vi "Configure.vi"(8 "error in":errorcluster, 10 "name":string="ePAS", 11 "ePAS in":refnum<class "ePAS.lvclass">) -> (0 "error out":errorcluster, 3 "ePAS out":refnum<class "ePAS.lvclass">)   [LabVIEW 2018, in "ePAS Library.lvlib" / "ePAS.lvclass"]
doc: "Configure the instrument class. If there is no config file specified, an error"
uses:
  ePAS.lvclass
  C:/Users/Labview/Documents/exscalabar_server/reusable/Instrument/Instrument.lvclass
  FPGA/Session/Exscalabar FPGA.lvclass
  C:/Program Files (x86)/National Instruments/LabVIEW 2018/user.lib/_Session Fwk/Session - Root.lvclass
  Commands/Change Laser Voffset/Change Laser Voffset.lvclass
  C:/Users/Labview/Documents/exscalabar_server/reusable/Command/Command.lvclass
  Commands/Change Laser Modulation/Change Laser Modulation.lvclass
  Commands/Change Laser Vrange/Change Laser Vrange.lvclass
  Commands/Change PAS Laser Frequency/Change Laser Frequency.lvclass
  Commands/Change Speaker State/Change Speaker State.lvclass
  Commands/Change Speaker Switch State/Change Speaker Switch State.lvclass
  Commands/Change iSpk Signal/Change iSpk Signal.lvclass
  Commands/Change Speaker Vparams/Change Speaker Vparams.lvclass
  Commands/Copy of Change Laser Enable State/Change Laser Enable State.lvclass
  reusable/Instrument/Instrument.lvclass/Instrument.ctl
  ePAS.lvclass/ePAS.ctl
  FPGA/Session/Exscalabar FPGA.lvclass/Exscalabar FPGA.ctl
  reusable/Session APIs/File Access/Config Data/Config Data.lvclass/Config Data.ctl
  Commands/Change Laser Voffset/Change Laser Voffset.lvclass/Change Laser Voffset.ctl
  Commands/Change Laser Vrange/Change Laser Vrange.lvclass/Change Laser Vrange.ctl
  Commands/Change PAS Laser Frequency/Change Laser Frequency.lvclass/Change Laser Frequency.ctl
  Commands/Copy of Change Laser Enable State/Change Laser Enable State.lvclass/Change Laser Enable State.ctl
  Commands/Change iSpk Signal/Change iSpk Signal.lvclass/Change iSpk Signal.ctl
  Commands/Change Speaker Switch State/Change Speaker Switch State.lvclass/Change Speaker Switch State.ctl
  Commands/Change Speaker Vparams/Change Speaker Vparams.lvclass/Change Speaker Vparams.ctl
  Commands/Change Laser Modulation/Change Laser Modulation.lvclass/Change Laser Modulation.ctl
  reusable/Session APIs/File Access/Config Data/Accessors/Read Ref.vi
  reusable/Instrument/Read Log Session.vi
  reusable/Instrument/Read Cfg Session.vi
  reusable/Instrument/Read CMD.vi
  Commands/Change Speaker Switch State/Write Length.vi
  Commands/Change Speaker Switch State/Write Period.vi
  Commands/Change Speaker Switch State/Write Cycle.vi
  FPGA/Session/Write logSession.vi
  FPGA/Session/Write configSession.vi
  reusable/Session APIs/File Access/Config Data/Config Data.lvclass
  reusable/Session APIs/File Access/Config Data/Read Array/Read Boolean Array.vi
  reusable/Session APIs/File Access/Config Data/Read Array/Read DBL Array.vi
  reusable/Session APIs/File Access/Config Data/Read Array/Read String Array.vi
  <vilib>/Utility/config.llb/Read Key (Boolean).vi
  <vilib>/Utility/config.llb/Read Key (I32).vi
  <vilib>/Utility/config.llb/Read Key (Double).vi
  reusable/PAS/Main/PAS.lvclass
  <userlib>/_Session Fwk/Session - Root.lvclass
  reusable/Command/Command.lvclass
  reusable/Session APIs/Session Log/System Log.lvclass
  <vilib>/Utility/config.llb/NI_LVConfig.lvlib
  <resource>/objmgr/daqmx.rc
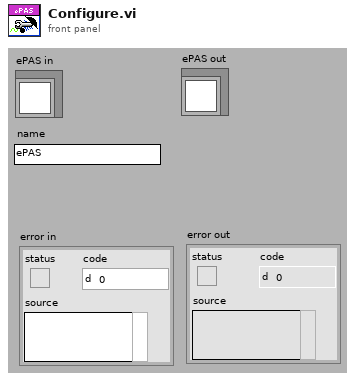
[diagram p1: front panel]
types:
  T1 = typedef "Session - Root.lvclass/Session Handle.ctl" = refnum<data-value>
  T2 = typedef "Config Data.lvclass/Config Session.ctl" = refnum<data-value>
  T3 = typedef "NI_LVConfig.lvlib/Config Data RefNum.ctl" = refnum<k1>
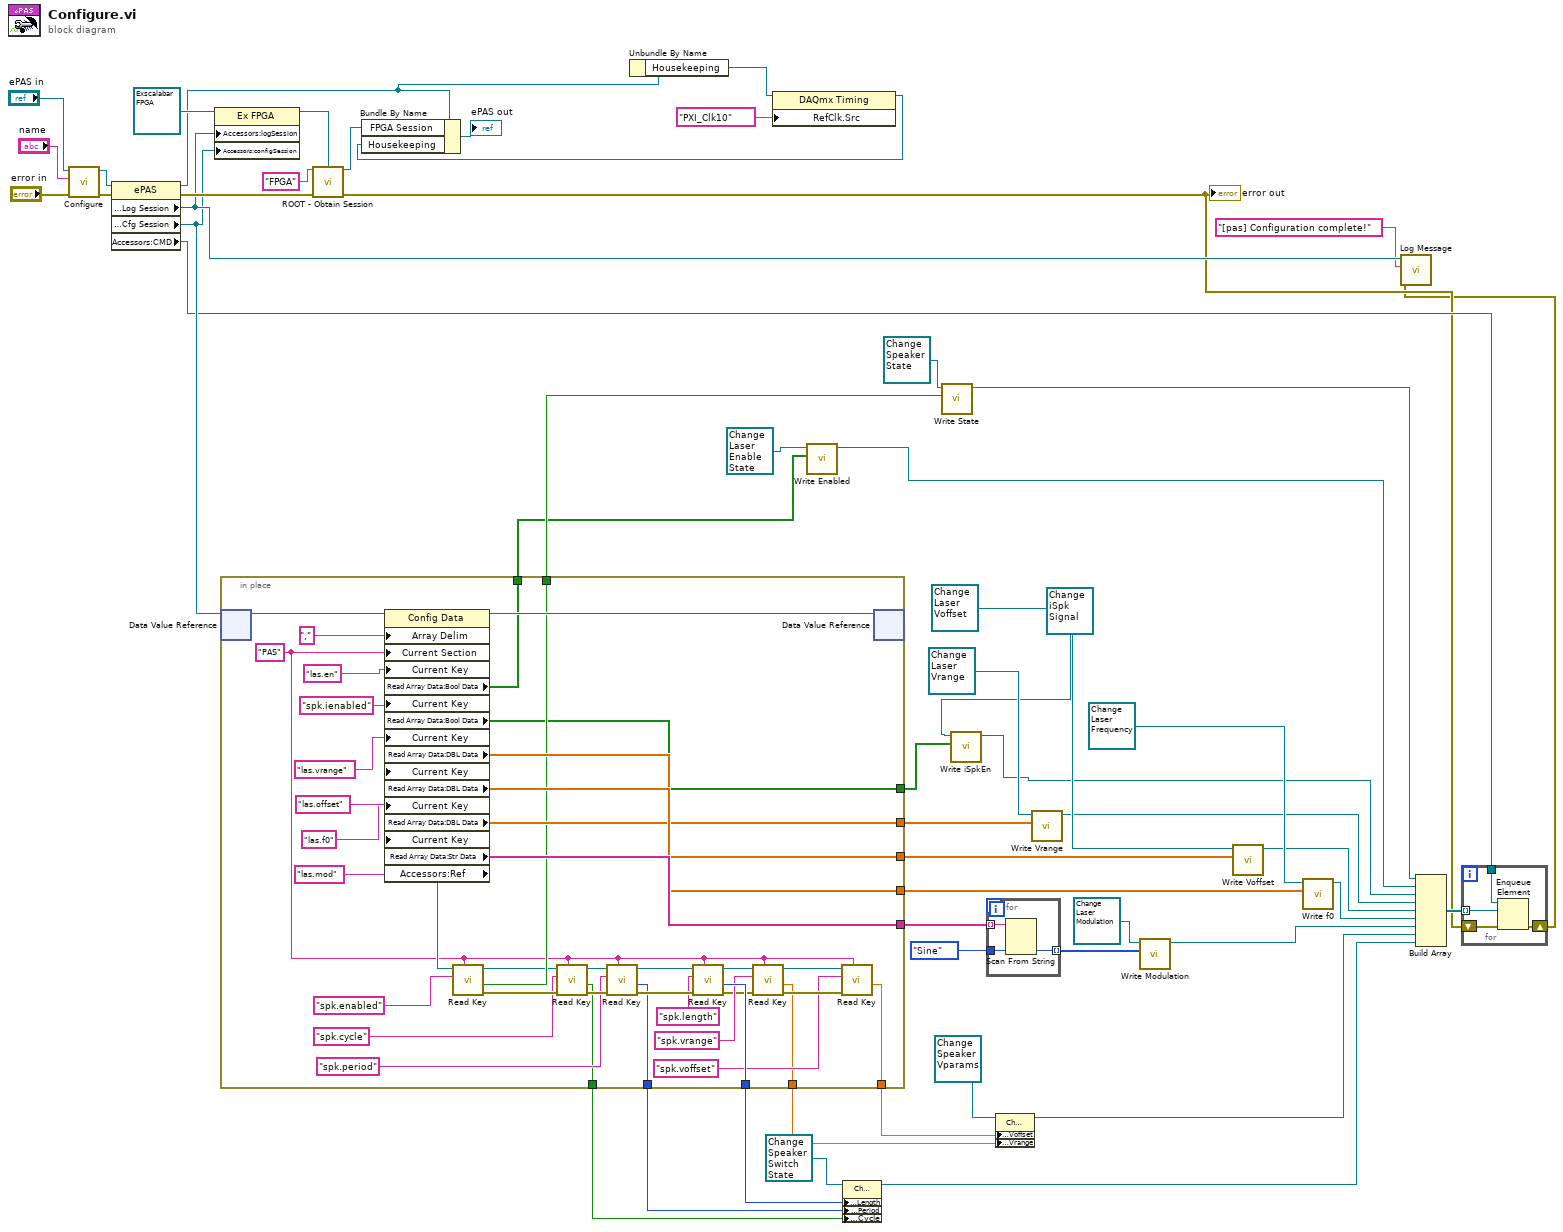
[diagram p0: block diagram]
diagram:
  n1 = call-parent "Configure.vi"("error in"="error in", "name"="name", "PAS in"="ePAS in") -> ("error out"=w44:errorcluster, "PAS out"=w50:refnum<class "ePAS.lvclass">)  [unwired: 7 in]
  n2 = property class="ePAS"(reference=w50, error in=w44) -> (reference out=w4:refnum<class "ePAS.lvclass">, error out=w45:errorcluster, "Accessors:Log Session"=w43:T1, "Accessors:Cfg Session"=w41:T2, "Accessors:CMD"=w32:refnum<queue>)
  n3 = property class="Ex FPGA"(reference=refnum<class "Exscalabar FPGA.lvclass"> refnum ("Ex FPGA"), "Accessors:logSession"=w43, "Accessors:configSession"=w41) -> (reference out=w48:refnum<class "Exscalabar FPGA.lvclass">)  [unwired: 1 in, 1 out]
  n4 = in-place {
    in-place-border: [w84] -> w40
    in-place-border: [w83] -> w24
    in-place-border: [w82] -> w36
    in-place-border: [w81] -> w33
    in-place-border: [w80] -> w7
    in-place-border: [w77] -> w29
    in-place-border: [w67] -> w27
    in-place-border: [w66] -> w23
    in-place-border: [w65] -> w26
    in-place-border: [w58] -> w21
    in-place-border: [w57] -> w22
    in-place-border: [w56] -> w13
    w60 = "PAS" ("Current Section")
    n5 = in-place-dvr #1(w41) -> (w93:refnum<class "Config Data.lvclass">)  [unwired: 1 out]
    n6 = property class="Config Data"(reference=w93, "Array Delim"=",", "Current Section"=w60, "Current Key"="las.en", "Current Key"="spk.ienabled", "Current Key"="las.vrange", "Current Key"="las.offset", "Current Key"="las.f0", "Current Key"="las.mod") -> (reference out=w89:refnum<class "Config Data.lvclass">, "Read Array Data:Bool Data"=w80:bool[], "Read Array Data:Bool Data"=w56:bool[], "Read Array Data:DBL Data"=w82:dbl[], "Read Array Data:DBL Data"=w83:dbl[], "Read Array Data:DBL Data"=w81:dbl[], "Read Array Data:Str Data"=w84:string[], "Accessors:Ref"=w79:T3)  [unwired: 1 in, 1 out]
    n7 = call-poly <vilib>:"Read Key.vi"("section"=w60, "key"="spk.enabled", "refnum"=w79) -> ("error out"=w75:errorcluster, "value"=w77:bool, "refnum out"=w76:T3)  [unwired: 5 in, 1 out]
    n8 = call-poly <vilib>:"Read Key.vi"("section"=w60, "error in (no error)"=w75, "key"="spk.cycle", "refnum"=w76) -> ("error out"=w73:errorcluster, "value"=w66:bool, "refnum out"=w74:T3)  [unwired: 4 in, 1 out]
    n9 = call-poly <vilib>:"Read Key.vi"("section"=w60, "error in (no error)"=w73, "key"="spk.period", "refnum"=w74) -> ("error out"=w71:errorcluster, "value"=w65:i32, "refnum out"=w72:T3)  [unwired: 4 in, 1 out]
    n10 = call-poly <vilib>:"Read Key.vi"("section"=w60, "error in (no error)"=w71, "key"="spk.length", "refnum"=w72) -> ("error out"=w55:errorcluster, "value"=w67:i32, "refnum out"=w64:T3)  [unwired: 4 in, 1 out]
    n11 = call-poly <vilib>:"Read Key.vi"("section"=w60, "error in (no error)"=w55, "key"="spk.vrange", "refnum"=w64) -> ("error out"=w61:errorcluster, "value"=w58:dbl, "refnum out"=w62:T3)  [unwired: 4 in, 1 out]
    n12 = call-poly <vilib>:"Read Key.vi"("section"=w60, "error in (no error)"=w61, "key"="spk.voffset", "refnum"=w62) -> ("value"=w57:dbl)  [unwired: 4 in, 3 out]
    n13 = in-place-dvr #1(w89) -> ()  [unwired: 2 out]
  }
  n14 = call <userlib>:"ROOT - Obtain Session.vi"("Session Name ()"="FPGA", "OBJ - Session"=w48, "error in (no error)"=w45) -> ("Session Handle"=w47:T1, "error out"=w6:errorcluster)  [unwired: 10 in, 1 out]
  "error out" <- w6
  n15 = Unbundle By Name(w4) -> ("Housekeeping"=w2:refnum<k21>)
  n16 = property class="DAQmx Timing"(reference=w2, "RefClk.Src"=tag "PXI_Clk10") -> (reference out=w1:refnum<k21>)  [unwired: 1 in, 1 out]
  n17 = Bundle By Name(cluster=w4, "FPGA Session"=w47, "Housekeeping"=w1) -> (→"ePAS out":refnum<class "ePAS.lvclass">)
  n18 = call "Write Enabled.vi"("Enabled?"=w7, "Change Laser Frequency in"=refnum<class "Change Laser Enable State.lvclass"> refnum ("ePAS Library.lvlib:Change Laser Enable State")) -> ("Change Laser Frequency out"=w8:refnum<class "Change Laser Enable State.lvclass">)  [unwired: 8 in, 1 out]
  n19 = property class="Change Speaker Switch"(reference=refnum<class "Change Speaker Switch State.lvclass"> refnum ("Change Speaker Switch"), "Accessors:Length"=w27, "Accessors:Period"=w26, "Accessors:Cycle"=w23) -> (reference out=w19:refnum<class "Change Speaker Switch State.lvclass">)  [unwired: 1 in, 1 out]
  n20 = call "Write State.vi"("State"=w29, "Change Speaker State in"=refnum<class "Change Speaker State.lvclass"> refnum ("Change Speaker State")) -> ("Change Speaker State out"=w14:refnum<class "Change Speaker State.lvclass">)  [unwired: 8 in, 1 out]
  n21 = call "Write iSpkEn.vi"("iSpkEn"=w13, "Change iSpkEn in"=refnum<class "Change iSpk Signal.lvclass"> refnum ("ePAS Library.lvlib:Change iSpk Signal.lvclass")) -> ("Change iSpkEn out"=w11:refnum<class "Change iSpk Signal.lvclass">)  [unwired: 8 in, 1 out]
  n22 = for {
    tunnel: w40 -> [w96] mode=indexing
    tunnel: [w95] -> w38 mode=indexing
    tunnel: enum8{"Sine", "Square"}."Sine" ("Mod") -> [w94]
    n23 = Scan From String(input string=w96, default 1=w94) -> (output 1=w95:enum8{"Sine", "Square"})  [unwired: 3 in, 3 out]
  }
  n24 = property class="Change Speaker Vparams"(reference=refnum<class "Change Speaker Vparams.lvclass"> refnum ("ePAS Library.lvlib:Change Speaker Vparams"), "Accessors:Voffset"=w22, "Accessors:Vrange"=w21) -> (reference out=w25:refnum<class "Change Speaker Vparams.lvclass">)  [unwired: 1 in, 1 out]
  n25 = call "Write Vrange.vi"("Vrange"=w36, "Change Laser Frequency in"=refnum<class "Change Laser Vrange.lvclass"> refnum) -> ("Change Laser Frequency out"=w15:refnum<class "Change Laser Vrange.lvclass">)  [unwired: 8 in, 1 out]
  n26 = call "Write Modulation.vi"("Modulation"=w38, "Change Laser Frequency in"=refnum<class "Change Laser Modulation.lvclass"> refnum) -> ("Change Laser Frequency out"=w18:refnum<class "Change Laser Modulation.lvclass">)  [unwired: 8 in, 1 out]
  n27 = call "Write Voffset.vi"("Voffset"=w24, "Change Laser Frequency in"=refnum<class "Change Laser Voffset.lvclass"> refnum ("Change Laser Voffset.lvclass")) -> ("Change Laser Frequency out"=w16:refnum<class "Change Laser Voffset.lvclass">)  [unwired: 8 in, 1 out]
  n28 = call "Write f0.vi"("f0"=w33, "Change Laser Frequency in"=refnum<class "Change Laser Frequency.lvclass"> refnum ("Change Laser Frequency.lvclass")) -> ("Change Laser Frequency out"=w17:refnum<class "Change Laser Frequency.lvclass">)  [unwired: 8 in, 1 out]
  n29 = Build Array(w14, w8, w11, w15, w16, w17, w18, w25, w19) -> (w31:refnum<class "Command.lvclass">[])
  n30 = for {
    tunnel: w32 -> [w100]
    tunnel: w31 -> [w99] mode=indexing
    shift-right: [w97] -> w5
    shift-left: w6 -> [w98]
    n31 = Enqueue Element(queue=w100, element=w99, error in (no error)=w98) -> (error out=w97:errorcluster)  [unwired: 1 in, 2 out]
  }
  n32 = call "Log Message.vi"("error in"=w5, "MSG In"="[pas] Configuration complete!", "session in"=w43) -> ()  [unwired: 7 in, 2 out]
